vi "trigger setting.vi"(8 "error in (no error)":errorcluster, 9 "Trigger Level (0.0 V)":dbl, 10 "Trigger Source (0: Channel 1)":u16(ring) items=["Channel 1", "Channel 2", "Channel 3", "Channel 4", "DIG 0", "DIG 1", "DIG 2", "DIG 3", "DIG 4", "DIG 5", "DIG 6", "DIG 7", "DIG 8", "DIG 9", "DIG 10", "DIG 11", "DIG 12", "DIG 13", "DIG 14", "DIG 15", "Line", "External"], 11 "OSC":refnum<visa-resource-name>) -> (0 "error out":errorcluster, 3 "OSC":refnum<visa-resource-name>)   [LabVIEW 2016]
uses:
  <instrlib>/Agilent 6000 Series/Public/Configure/Configure Edge Trigger Source.vi
  <instrlib>/Agilent 6000 Series/Agilent 6000 Series.lvlib
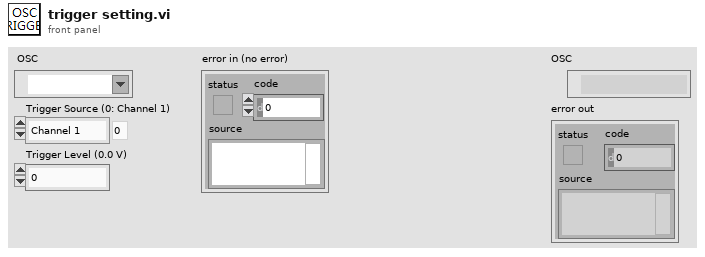
[diagram p1: front panel]
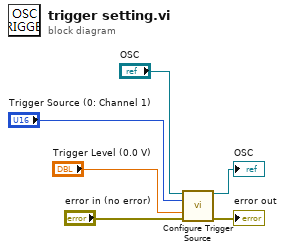
[diagram p0: block diagram]
diagram:
  n1 = call-poly <instrlib>:"Configure Trigger Source.vi"("VISA resource name"="OSC", "Trigger Source (0: Channel 1)"="Trigger Source (0: Channel 1)", "Trigger Level (0.0 V)"="Trigger Level (0.0 V)", "error in (no error)"="error in (no error)") -> ("VISA resource name out"=→"OSC":refnum<visa-resource-name>, "error out"=→"error out":errorcluster)  [unwired: 10 in]
